vi "Stepper Music Code.vi"() -> ()   [LabVIEW 2014]
uses:
  <vilib>/LabVIEW Targets/FPGA/cRIO/cRIO-9505/controls.llb/_nicrio_cRIO-9505_DriveStatus.ctl
  <vilib>/FPGAPlugInAG/cRIO-9074/niLvFpga_Open_cRIO-9074.vi
  <vilib>/Utility/error.llb/Error Cluster From Error Code.vi
  <vilib>/rvi/errors/niLvFpgaAdjustHostInterfaceError.vi
  <vilib>/FPGAPlugInAG/cRIO-9074/niLvFpga_Close_cRIO-9074.vi
  <vilib>/rvi/interface/nirviOpenFPGA/nirviOpenFPGA.xnode
  FPGA Bitfiles/MotorLabAProject_FPGATarget_fullfpgalayer_geeQA2EZIvY.lvbitx
  full_fpga_layer.vi
  <vilib>/rvi/interface/nirviReadWriteControl/nirviReadWriteControl.xnode
  <vilib>/rvi/interface/nirviCloseFPGA/nirviCloseFPGA.xnode
  NiFpgaLv.dll
panel:
  out "Total Loop Count":i32
  out "Step period \ncommand (Note)":i32
  out "For Loop Counter":i32
  out "Step Command\n(Duration)":i32
  out "Duration":i32[](array[numeric])
  out "Note":i32[](array[numeric])
  in  "Stepper Step Period (uS)":i16
  out "VI IS RUNNING":bool
  in  "Desired Position (Steps)":i32
  out "error out":errorcluster
  in  "stop":bool
  in  "Reset Stepper Counter":bool
  out "Stepper Steps to move":i32
  out "Stepper Current (Steps)":i32
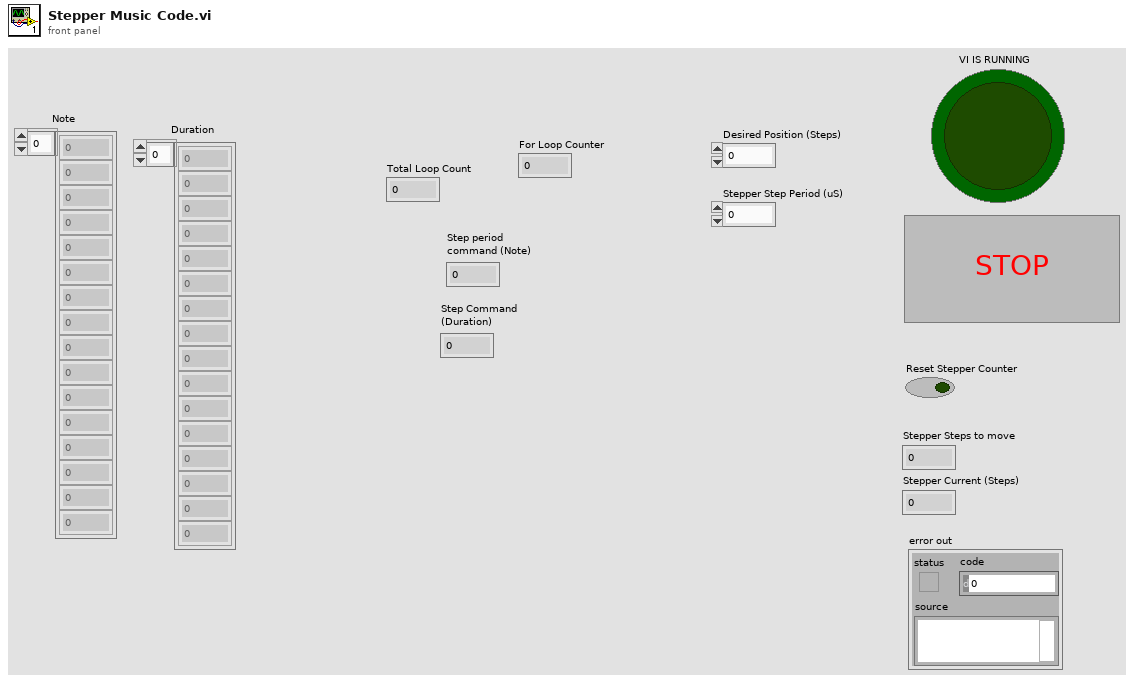
[diagram p1: front panel]
types:
  T1 = typedef "_nicrio_cRIO-9505_DriveStatus.ctl" = enum8{"Enabled", "Disabled", "Disabled by Drive Fault", "Disabled by Temp. Fault", "Disabled by E-Stop", "Unknown"}
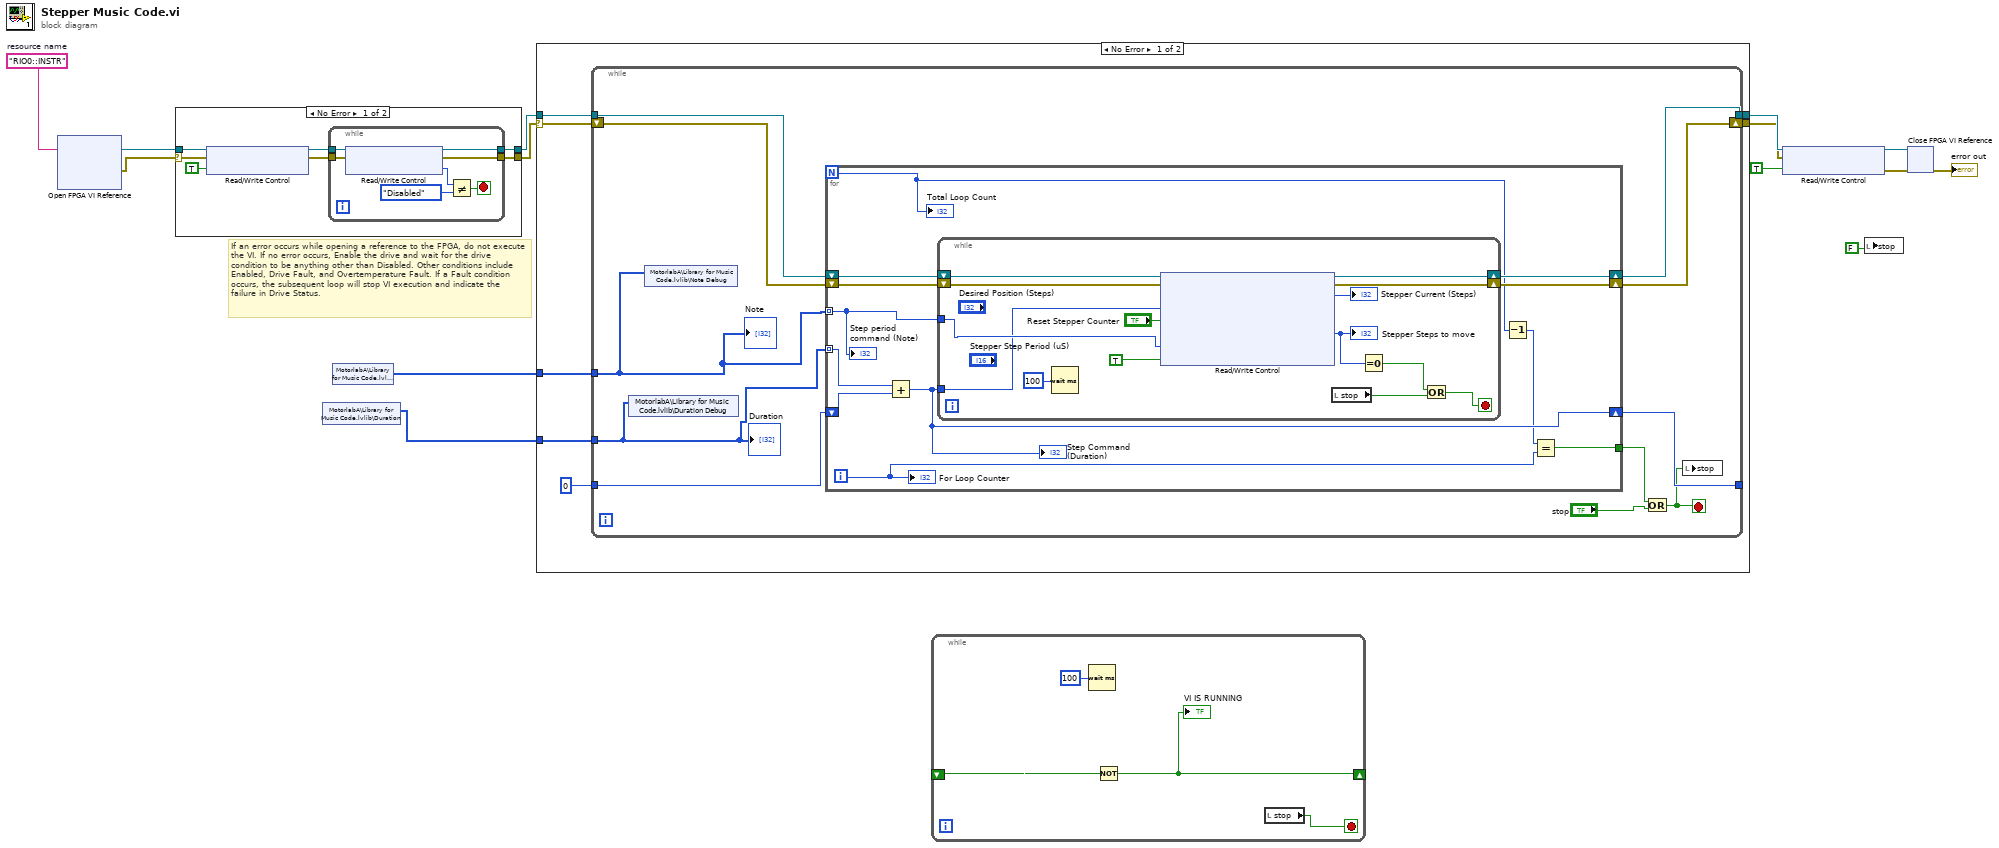
[diagram p0: block diagram]
diagram:
  w5 = "RIO0::INSTR"  # resource name
  # "If an error occurs while opening a reference to the FPGA, do not execute the VI. If no error occurs, Enable the drive and wait for the drive condition to be anything other than Disabled. Other conditions include Enabled, Drive Fault, and Overtemperature Fault. If a Fault condition occurs, the subsequent loop will stop VI execution and indicate the failure in Drive Status."
  n1 = xnode "Open FPGA VI Reference"("resource name"=w5) -> ("FPGA VI Reference Out"=w8:refnum<k20>, "error out"=w7:errorcluster)  [unwired: 1 in]
  n2 = case shown="No Error" w7 {
    selector: w7 -> [w16 w29]
    tunnel: w8 -> [w19 w30]
    tunnel: [w21 w30] -> w9
    tunnel: [w20 w29] -> w6
    frame No Error {
      n3 = xnode "Read/Write Control"("FPGA VI Reference In"=w19, "error in"=w16, "PWM  Enable Drive"=TRUE ("Enable Drive")) -> ("FPGA VI Reference Out"=w18:refnum<k20>, "error out"=w17:errorcluster)
      n4 = while {
        tunnel: [w28] -> w21
        tunnel: [w24] -> w20
        tunnel: w18 -> [w23]
        tunnel: w17 -> [w22]
        stop <- w25 stop-if-true
        n5 = xnode "Read/Write Control"("FPGA VI Reference In"=w23, "error in"=w22) -> ("FPGA VI Reference Out"=w28:refnum<k20>, "error out"=w24:errorcluster, "PWM Drive Status"=w27:T1)
        n6 = Not Equal?(x=w27, y=_nicrio_cRIO-9505_DriveStatus."Disabled") -> (x != y?=w25:bool)
      }
    }
    frame Error {
      # "Error occurred. Do not run."
    }
  }
  n7 = shared-variable "MotorlabA\\Library for Music Code.lvlib\\Duration"() -> (w1:i32[])  [unwired: 1 in, 1 out]
  n8 = shared-variable "MotorlabA\\Library for Music Code.lvlib\\Note"() -> (w2:i32[])  [unwired: 1 in, 1 out]
  n9 = case shown="No Error" w6 {
    selector: w6 -> [w35 w75]
    tunnel: w9 -> [w37 w76]
    tunnel: [w34 w76] -> w14
    tunnel: [w36 w75] -> w13
    tunnel: w2 -> [w33 _]
    tunnel: w1 -> [w32 _]
    frame No Error {
      n10 = while {
        tunnel: w37 -> [w48]
        shift-right: [w46] -> w36
        shift-left: w35 -> [w47]
        tunnel: [w45] -> w34
        tunnel: w33 -> [w44]
        tunnel: w32 -> [w43]
        tunnel: 0 -> [w41]
        tunnel: [w42] -> _
        stop <- w38 stop-if-true
        n11 = shared-variable "MotorlabA\\Library for Music Code.lvlib\\Duration Debug"(w43) -> ()  [unwired: 1 in, 1 out]
        n12 = shared-variable "MotorlabA\\Library for Music Code.lvlib\\Note Debug"(w44) -> ()  [unwired: 1 in, 1 out]
        n13 = for {
          N -> [w51]
          shift-right: [w57] -> w45
          shift-left: w48 -> [w60]
          shift-right: [w58] -> w46
          shift-left: w47 -> [w59]
          tunnel: w44 -> [w53] mode=indexing
          tunnel: w43 -> [w56] mode=indexing
          shift-right: [w54] -> w42
          shift-left: w41 -> [w55]
          tunnel: [w49] -> w39
          i -> [w52]
          n14 = Add(x=w56, y=w55) -> (x+y=w54:i32)
          "Step Command\n(Duration)" <- w54
          n15 = while {
            tunnel: w53 -> [w64]
            shift-right: [w68] -> w57
            shift-left: w60 -> [w71]
            shift-right: [w69] -> w58
            shift-left: w59 -> [w70]
            tunnel: w54 -> [w63]
            stop <- w67 stop-if-true
            n16 = Wait (ms)(milliseconds to wait=u32 100) -> ()  [unwired: 1 out]
            n17 = xnode "Read/Write Control"("FPGA VI Reference In"=w71, "error in"=w70, "Stepper Desired Position (Steps)"=w63, "Stepper Reset Step Counter"="Reset Stepper Counter", "Stepper  Step Period (uS)"=w64, "Stepper Enable/Disable Step Motor"=TRUE) -> ("FPGA VI Reference Out"=w68:refnum<k20>, "error out"=w69:errorcluster, "Stepper Current (Steps)"=→"Stepper Current (Steps)":i32, "Stepper Steps to move"=w62:i32)
            "Stepper Steps to move" <- w62
            n18 = local read "stop"() -> (w65:bool)
            n19 = Equal To 0?(x=w62) -> (x = 0?=w66:bool)
            n20 = Or(x=w66, y=w65) -> (x .or. y?=w67:bool)
          }
          n21 = Decrement(x=w51) -> (x-1=w50:i32)
          n22 = Equal?(x=w50, y=w52) -> (x = y?=w49:bool)
          "For Loop Counter" <- w52
          "Step period \ncommand (Note)" <- w53
          "Total Loop Count" <- w51
        }
        n23 = Or(x=w39, y="stop") -> (x .or. y?=w38:bool)
        n24 = local write "stop"(w38) -> ()
        "Note" <- w44
        "Duration" <- w43
      }
    }
    frame Error {
      # "Error occurred. Do not run."
    }
  }
  n25 = while {
    shift-right: [w78] -> _
    shift-left: _ -> [w79]
    stop <- w80 stop-if-true
    n26 = Wait (ms)(milliseconds to wait=u32 100) -> ()  [unwired: 1 out]
    n27 = Not(x=w79) -> (.not. x?=w78:bool)
    "VI IS RUNNING" <- w78
    n28 = local read "stop"() -> (w80:bool)
  }
  n29 = xnode "Read/Write Control"("FPGA VI Reference In"=w14, "error in"=w13, "PWM Disable Drive"=TRUE ("Disable Drive")) -> ("FPGA VI Reference Out"=w12:refnum<k20>, "error out"=w11:errorcluster)
  n30 = local write "stop"(FALSE) -> ()
  n31 = xnode "Close FPGA VI Reference"("FPGA VI Reference In"=w12, "error in"=w11) -> ("error out"=→"error out":errorcluster)
